vi "Do.vi"(8 "error in (no error)":errorcluster, 10 "Actor in":refnum<class "Actor.lvclass">, 11 "Reply Message":refnum<class "Iterator Reply Msg.lvclass">) -> (0 "error out":errorcluster, 2 "Actor out":refnum<class "Actor.lvclass">)   [LabVIEW 2016, in "Iterator Actor.lvlib" / "Iterator Reply Msg.lvclass"]
doc: "Launches the dynamic dispatch Do Core.vi method, writes until it finishes, and returns its Boolean reply to the queue defined in Send Message and Wait For Responce.vi method.\n\nThe error of the Enqueue Element method is erased to not stop the action of the Caller actor. Nevertheless, this error will be reported by the Iterator actor, and should be processed by the Caller."
uses:
  Iterator Reply Msg.lvclass
  <vilib>/ActorFramework/Actor/Actor.lvclass
  Iterator Reply Msg.lvclass/Iterator Reply Msg.ctl
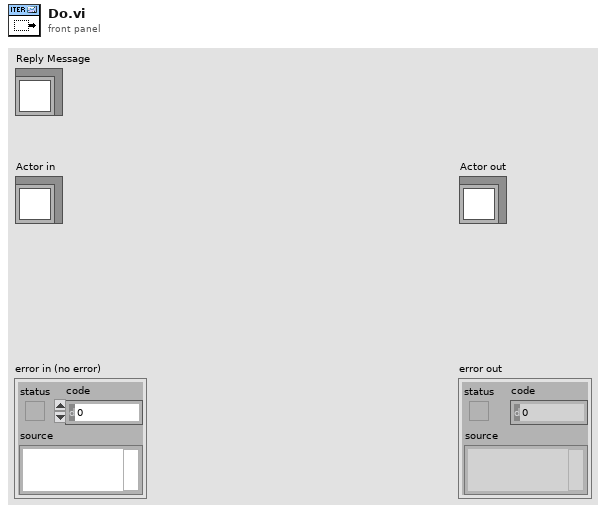
[diagram p1: front panel]
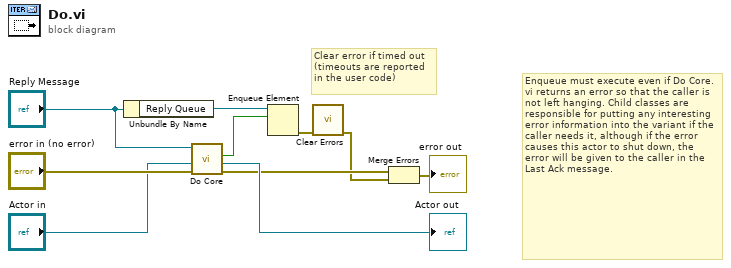
[diagram p0: block diagram]
diagram:
  # "Clear error if timed out\n(timeouts are reported \nin the user code)"
  # "Enqueue must execute even if Do Core.vi returns an error so that the caller is not left hanging. Child classes are responsible for putting any interesting error information into the variant if the caller needs it, although if the error causes this actor to shut down, the error will be given to the caller in the Last Ack message."
  n1 = Unbundle By Name("Reply Message") -> ("Reply Queue"=w6:refnum<queue>)
  n2 = call-dynamic "Do Core.vi"("error in (no error)"="error in (no error)", "Actor in"="Actor in", "Reply Message"="Reply Message") -> ("error out"=w3:errorcluster, "Actor out"=→"Actor out":refnum<class "Actor.lvclass">, "Reply"=w5:bool)  [unwired: 6 in]
  n3 = Enqueue Element(queue=w6, element=w5) -> (error out=w2:errorcluster)  [unwired: 2 in, 2 out]
  n4 = call <vilib>:"Clear Errors.vi"("error in (no error)"=w2) -> ("error out"=w1:errorcluster)  [unwired: 5 in, 1 out]
  n5 = Merge Errors(w3, w1) -> (→"error out":errorcluster)
